vi "art联动采集V4.2.vi"() -> ()   [LabVIEW 2016]
uses:
  <vilib>/Instr/_visa.llb/VISA Configure Serial Port (Instr).vi
  <vilib>/Utility/file.llb/Write Delimited Spreadsheet (DBL).vi
panel:
  in  "定位模式":bool
  in  "X终点":dbl
  in  "Y终点":dbl
  in  "高级设置":bool
  in  "Y轴回零速度":dbl=15000.0
  in  "X轴回零速度":dbl=15000.0
  in  "细分设置":dbl=8.0
  in  "等待时间":u32=40
  in  "文件保存":path=path "C:/Users/H301/Desktop/art采集实验数据" caption="保存路径"
  out "行用时（s）":dbl
  out "time（行）":u32
  out "hDevice out":i32=253955776
  out "error out":errorcluster caption="错误输出"
  in  "退出扫描(Esc)":bool
  out "N_Length":i32=16384
  out "M_Length":i32
  out "hDevice":i32=241832032
  out "pulDDR2Length":u32=256
  out "总用时（s）":dbl
  out "毫秒计时值":u32=3586537
  out "数组":dbl[][](array[numeric])=[[58819.77200735986, 88200.32943600747]]
  out "强度图":dbl[][](graph)=[[58819.77200735986, 88200.32943600747]]
  out "judge":dbl
  out "Xloop":dbl
  out "幅频谱":dbl[](graph)
  out "时域谱":dbl[](graph)
  out "错误输出":errorcluster
  in  "启动":bool
  in  "开始扫描":bool
  in  "X归零":bool
  in  "Y归零":bool
  in  "Y起点":dbl
  in  "Y轴速度":dbl=9000.0
  in  "X轴速度":dbl=9000.0
  out "电机状态":bool
  in  "电机端口":refnum<visa-resource-name>="COM6"
  out "Yloop":dbl=1.0
  out "X扫描范围":dbl=150.0
  out "Y扫描范围":dbl=75.0
  out "Y序":i32
  in  "X起点":dbl
  out "Y(mm)":dbl
  out "x+y 2":dbl=3.0
  in  "Y步进":dbl=1.0
  in  "精度":dbl=0.001
  in  "电机急停":bool
  out "X（mm）":dbl
  out "x+y":dbl=1.0
  in  "X步进":dbl=1.0
  # "实时坐标"
  # "时域谱"
  # "频域谱"
  # "扫描参数"
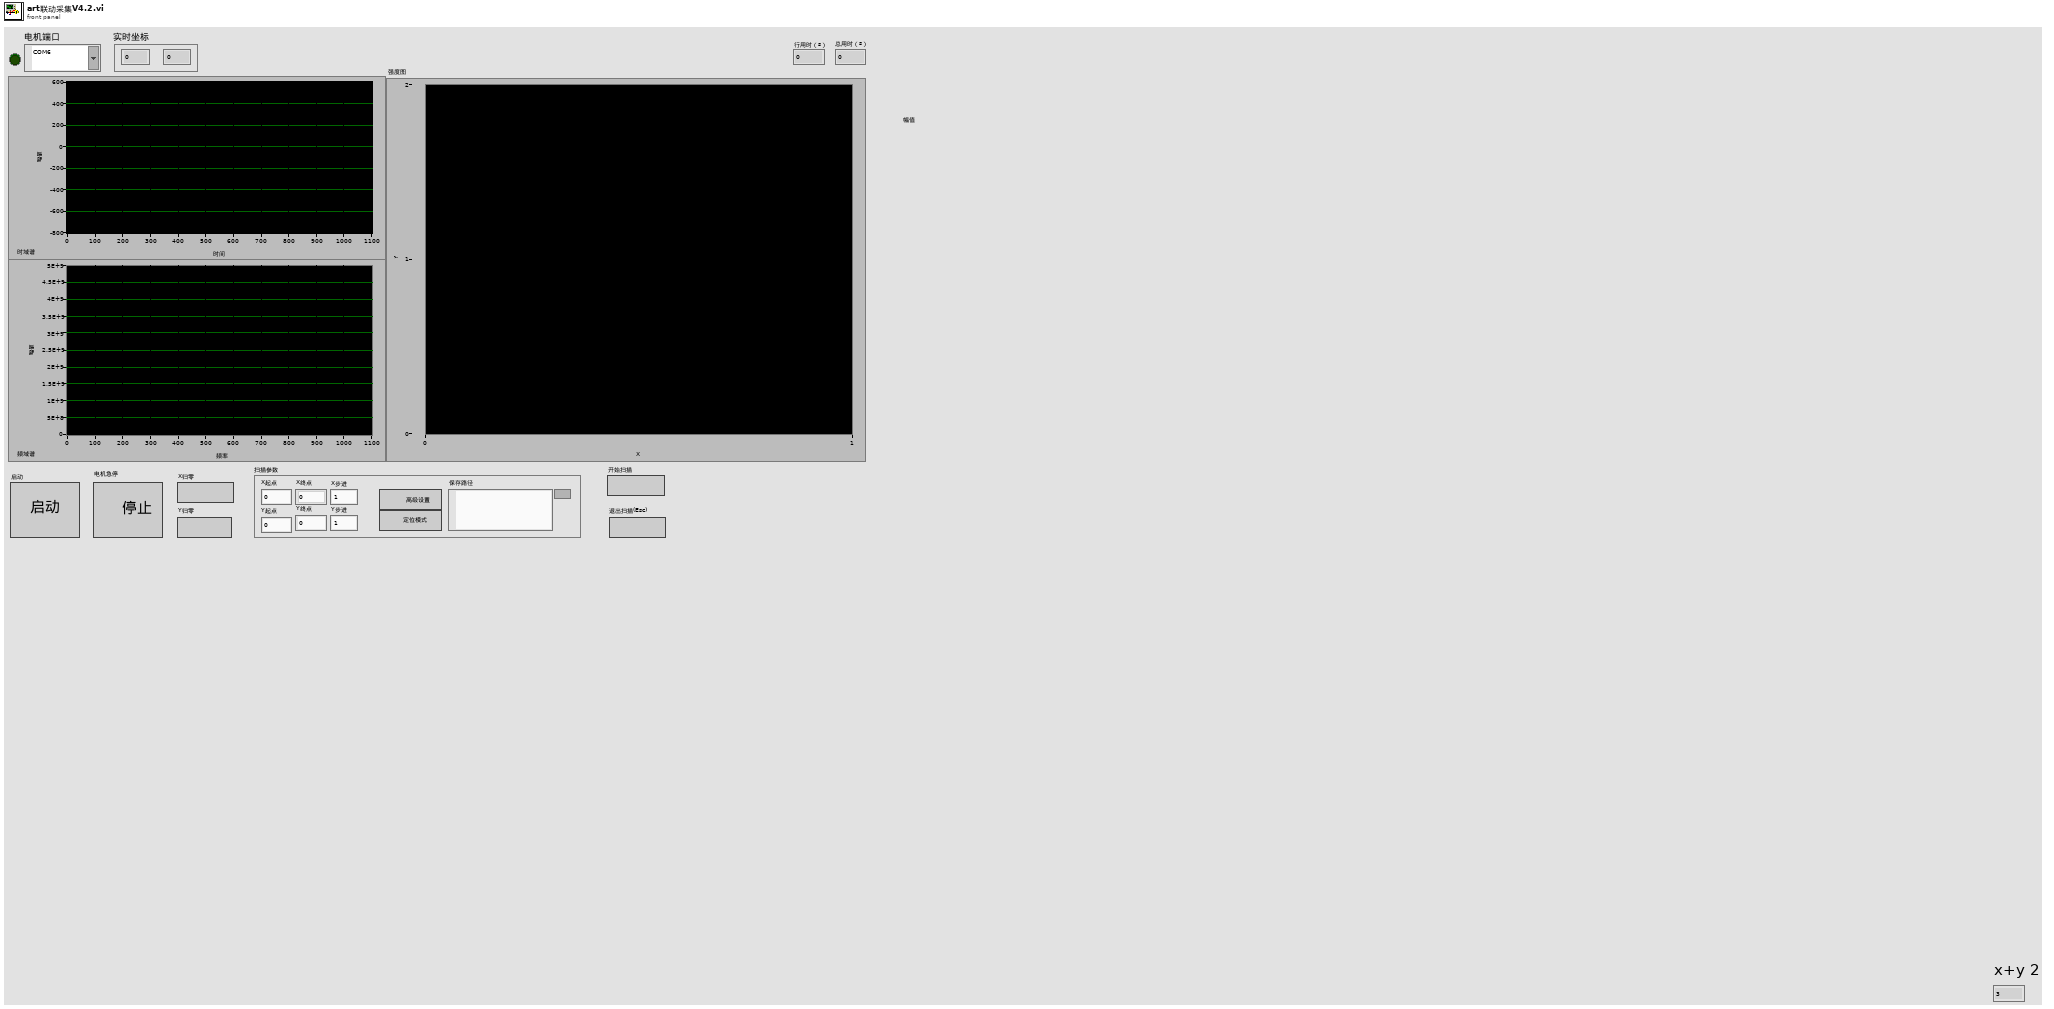
[diagram p1: front panel]
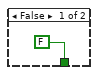
[diagram p2: hidden frame]
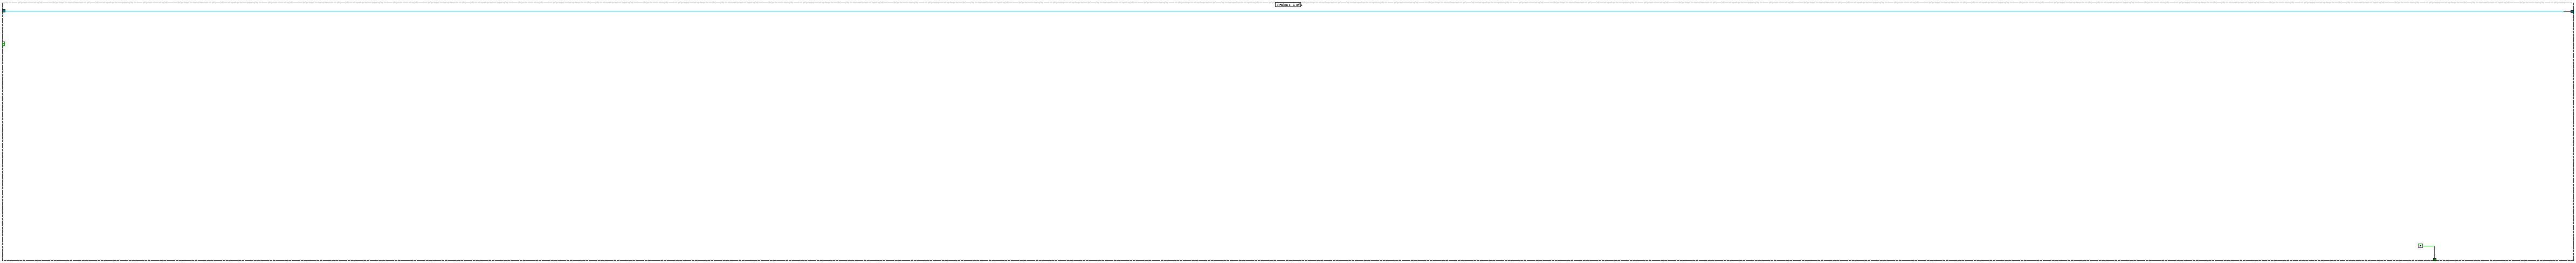
[diagram p3: hidden frame]
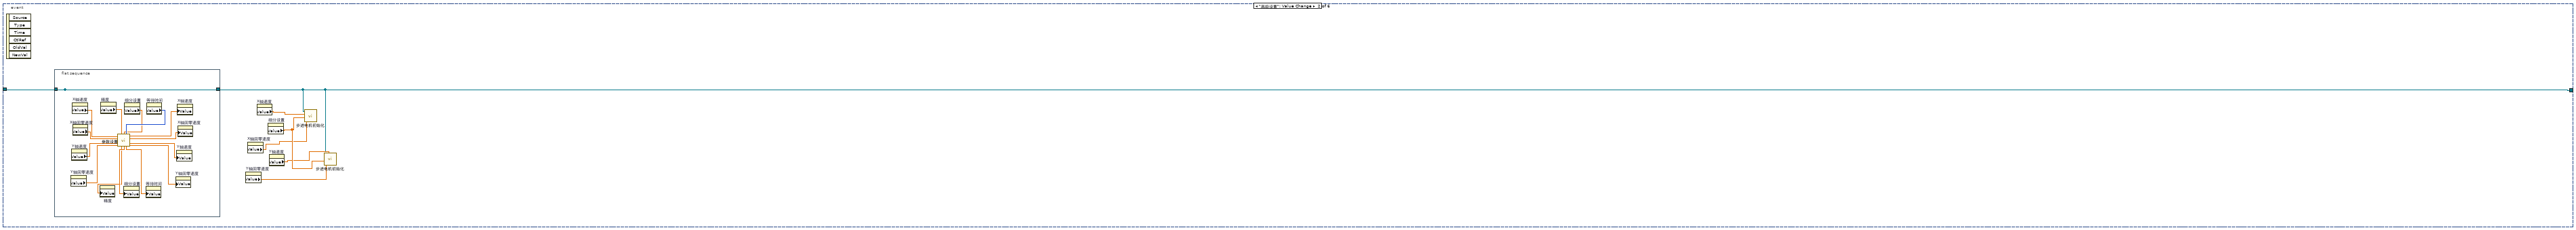
[diagram p4: hidden frame]
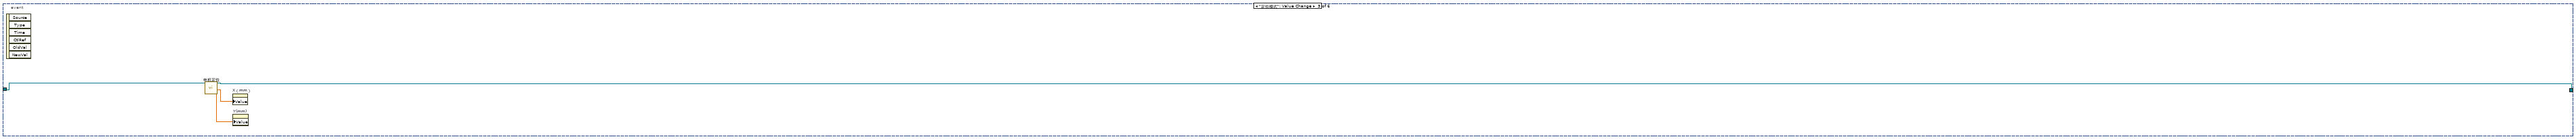
[diagram p5: hidden frame]
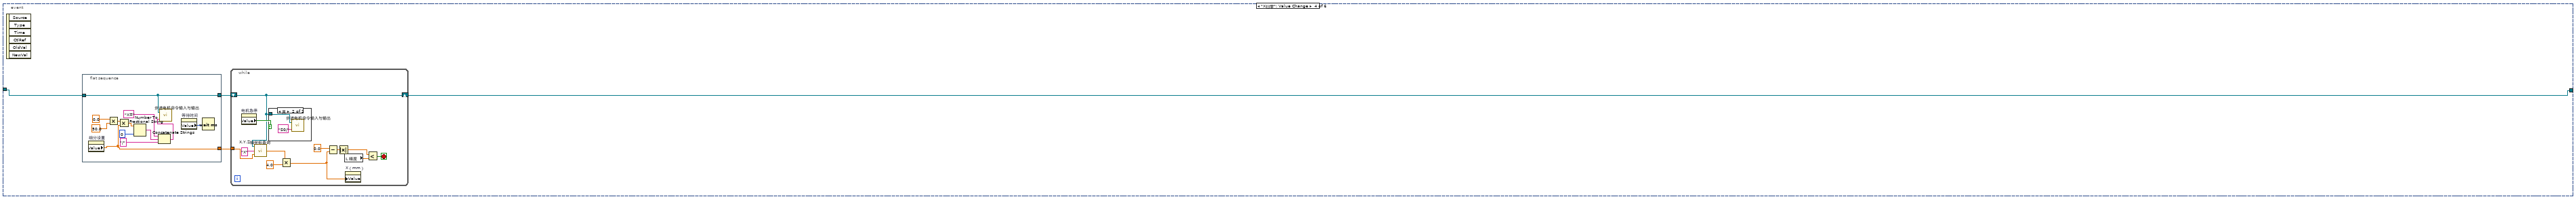
[diagram p6: hidden frame]
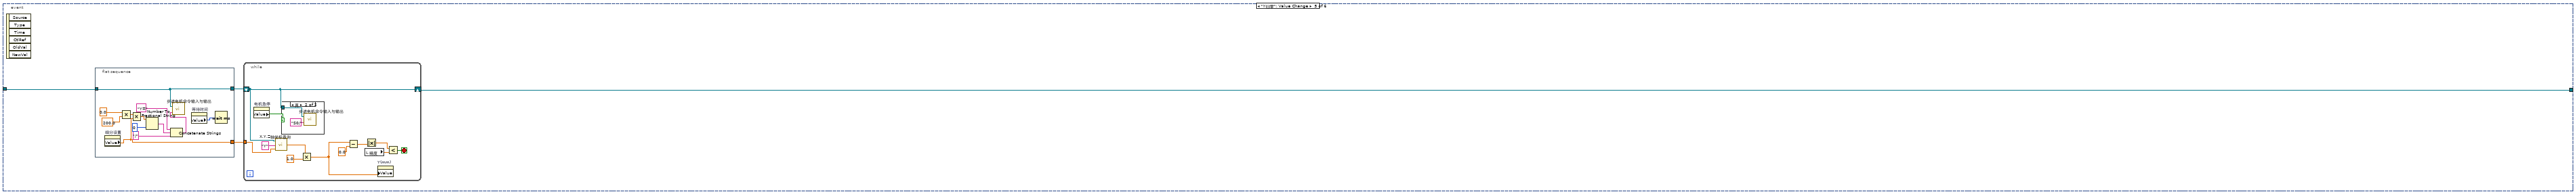
[diagram p8: hidden frame]
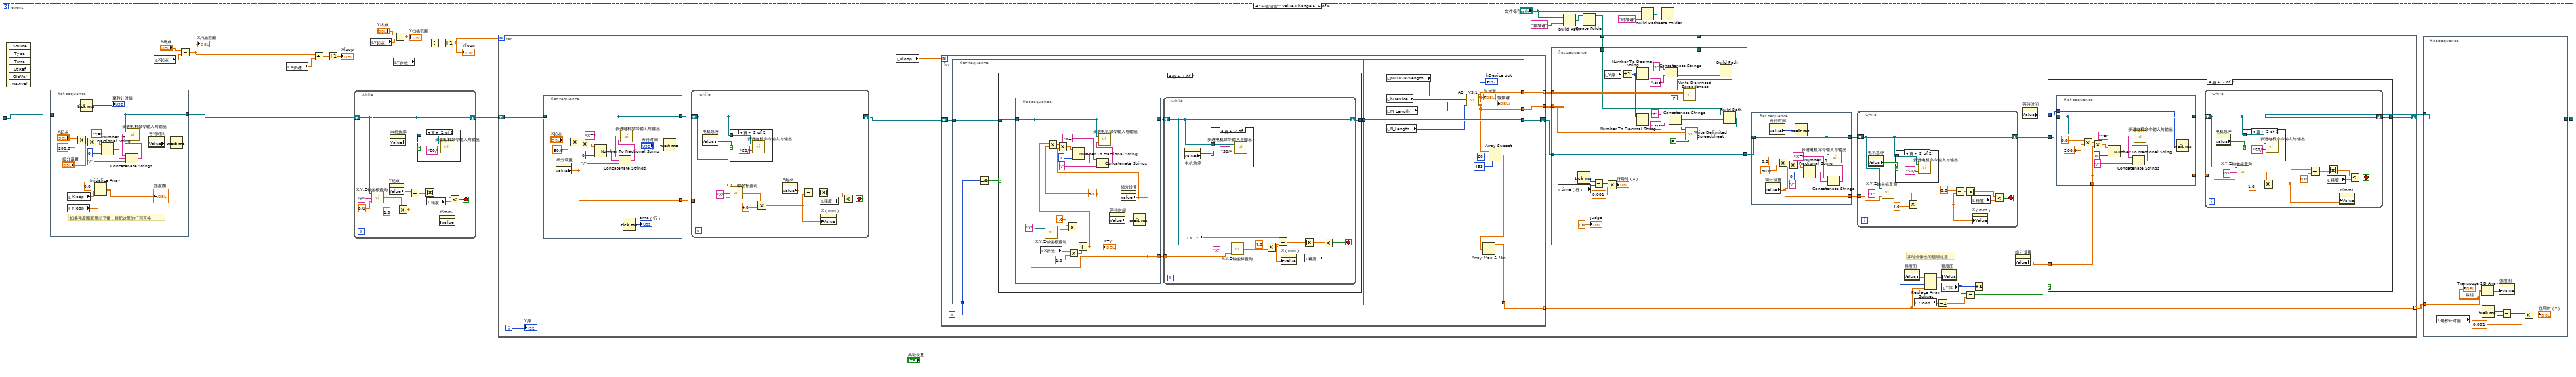
[diagram p10: hidden frame]
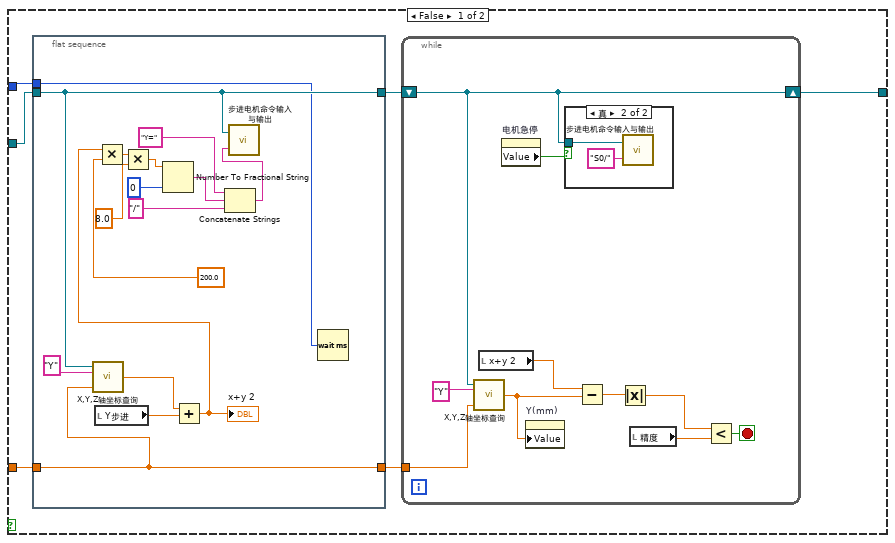
[diagram p14: hidden frame]
diagram:
  n1 = while {
    stop <- w3 stop-if-true
    n2 = case shown="真" "启动" {
      tunnel: [FALSE ("ESC") w10] -> w3
      frame False {
      }
      frame True {
        w25 = 0  # OutClockSource
        w26 = 0  # bClockSourceDir
        w28 = 10000000  # Frequency
        w29 = 0  # ClockSource
        w30 = 0  # TrigLevelVolt
        w17 = 1
        w31 = 0  # TriggerDir
        w32 = 0  # TriggerSource
        w33 = 0  # ATRTriggerChannel
        w34 = 0  # TriggerMode
        w18 = 4096  # N_Length
        w19 = 0  # M_Length
        w35 = 1  # CouplingType
        w36 = 0  # DeviceLgcID
        w46 = u16 0 items=["无", "XON/XOFF", "RTS/CTS", "XON/XOFF & RTS/CTS", "DTR/DSR", "XON/XOFF & DTR/DSR"] ("flow control (0:none)")
        w47 = u16 10 items=["1.0"=10, "1.5"=15, "2.0"=20] ("stop bits (10: 1 bit)")
        # "3"
        # "2"
        # "1"
        n3 = call-poly "VISA Configure Serial Port"("VISA resource name"="电机端口", "baud rate (9600)"=u32 9600, "data bits (8)"=u16 8, "parity (0:none)"=enum16{"None", "Odd", "Even", "Mark", "Space"}."None", "stop bits (10: 1 bit)"=w47, "flow control (0:none)"=w46) -> ("VISA resource name out"=w38:refnum<visa-resource-name>, "error out"=→"error out":errorcluster)  [unwired: 1 in, 7 out]
        n4 = Build Array "InputRange"(w17, w17, w17, w17) -> (w16:i32[])
        n5 = dll-call lib="PTH2aabs CUsersH301Desktopart闭环扫描程序采集卡控制INFamd64PCI8502_32.dll" fn="PCI8502_CreateDevice" label="CreateDevice"("DeviceLgcID"=w36) -> (w23:i32)  [unwired: 4 in, 2 out]
        n6 = property on="细分设置" class="DigNum (严格)"() -> ("Value"=w9:dbl)  [unwired: 2 in, 2 out]
        n7 = Build Array (concatenate) "InitDeviceAD"(w28, w16, w35, w19, w18, w34, w33, w32, w31, w30, w29, w26, w25) -> (w27:i32[])
        n8 = call "步进电机初始化.vi"("回零速度"="X轴回零速度", "细分设置"=w9, "X轴速度"="X轴速度", "串口通信端口"=w38) -> ()  [unwired: 2 in, 1 out]
        n9 = dll-call lib="PTH2aabs CUsersH301Desktopart闭环扫描程序采集卡控制INFamd64PCI8502_32.dll" fn="PCI8502_GetDDR2Length" label="GetDDR2Length"("hDevice"=w23, "pulDDR2Length"=u32 0) -> ("hDevice"=w22:i32, "pulDDR2Length"=→"pulDDR2Length":u32)  [unwired: 4 in, 2 out]
        n10 = call "步进电机初始化.vi"("Y轴速度"="Y轴速度", "回零速度"="Y轴回零速度", "细分设置"=w9, "串口通信端口"=w38) -> ()  [unwired: 2 in, 1 out]
        n11 = call "步进电机命令输入与输出.vi"("输入字符串"="?R/", "串口通信端口"=w38) -> ("返回字符串"=w43:string)
        n12 = dll-call lib="PTH2aabs CUsersH301Desktopart闭环扫描程序采集卡控制INFamd64PCI8502_32.dll" fn="PCI8502_InitDeviceAD" label="InitDeviceAD"("hDevice"=w22, "pADPara"=w27) -> ("hDevice"=→"hDevice":i32)  [unwired: 5 in, 2 out]
        n13 = String Subset(string=w43, offset (0)=0 ("偏移量(0)"), length (rest)=2 ("长度（剩余）")) -> (substring=w40:string)
        n14 = Equal?(x=w40, y="OK") -> (x = y?=w37:bool)
        "电机状态" <- w37
        n15 = case shown="真" w37 {
          tunnel: w38 -> [w53 w56]
          tunnel: [w53 w54] -> w11
          tunnel: [FALSE ("ESC") w55] -> w10
          frame False {
          }
          frame True {
            n16 = while {
              tunnel: ["退出扫描(Esc)"] -> w55
              shift-right: [w57] -> w54
              shift-left: w56 -> [w62]
              stop <- "退出扫描(Esc)" stop-if-true
              n17 = property on="高级设置" class="Bool"("Visible"=TRUE ("可见")) -> ()  [unwired: 2 in, 2 out]
              n18 = property on="定位模式" class="Bool"("Visible"=TRUE ("可见")) -> ()  [unwired: 2 in, 2 out]
              n19 = event shown="[0] 超时" {
                selector: _ -> [_ _ _ _ _ _]
                dyn-events: _ -> [_ _ _ _ _ _]
                timeout: 1 -> [_ _ _ _ _ _]
                tunnel: w62 -> [w63 w70 w89 w93 w123 w174]
                tunnel: [w63 w64 w88 w91 w121 w168] -> w57
                event Timeout {
                  n20 = event-data() -> ()  [unwired: 1 in, 3 out]
                }
                event "高级设置": Value Change {
                  n21 = event-data() -> ()  [unwired: 1 in, 6 out]
                  n22 = flat-sequence {
                    tunnel: w70 -> [w71]
                    tunnel: [w71] -> _
                    tunnel: [w71] -> w64
                    frame #0 {
                      n23 = property on="Y轴回零速度" class="DigNum (严格)"() -> ("Value"=w75:dbl)  [unwired: 2 in, 2 out]
                      n24 = property on="Y轴速度" class="DigNum (严格)"() -> ("Value"=w74:dbl)  [unwired: 2 in, 2 out]
                      n25 = property on="X轴速度" class="DigNum (严格)"() -> ("Value"=w72:dbl)  [unwired: 2 in, 2 out]
                      n26 = property on="X轴回零速度" class="DigNum (严格)"() -> ("Value"=w73:dbl)  [unwired: 2 in, 2 out]
                      n27 = property on="精度" class="DigNum (严格)"() -> ("Value"=w79:dbl)  [unwired: 2 in, 2 out]
                      n28 = property on="细分设置" class="DigNum (严格)"() -> ("Value"=w80:dbl)  [unwired: 2 in, 2 out]
                      n29 = property on="等待时间" class="DigNum (严格)"() -> ("Value"=w81:u32)  [unwired: 2 in, 2 out]
                      n30 = call "参数设置.vi"("X轴速度"=w72, "精度"=w79, "细分设置"=w80, "等待时间"=w81, "X轴回零速度"=w73, "Y轴速度"=w74, "Y轴回零速度"=w75) -> ("X轴速度"=w82:dbl, "X轴回零速度"=w83:dbl, "Y轴速度"=w84:dbl, "精度"=w76:dbl, "细分设置"=w77:dbl, "等待时间"=w78:dbl, "Y轴回零速度"=w85:dbl)  [unwired: 2 in]
                      n31 = property on="精度" class="DigNum (严格)"("Value"=w76) -> ()  [unwired: 2 in, 2 out]
                      n32 = property on="细分设置" class="DigNum (严格)"("Value"=w77) -> ()  [unwired: 2 in, 2 out]
                      n33 = property on="等待时间" class="DigNum (严格)"("Value"=w78) -> ()  [unwired: 2 in, 2 out]
                      n34 = property on="Y轴回零速度" class="DigNum (严格)"("Value"=w85) -> ()  [unwired: 2 in, 2 out]
                      n35 = property on="Y轴速度" class="DigNum (严格)"("Value"=w84) -> ()  [unwired: 2 in, 2 out]
                      n36 = property on="X轴速度" class="DigNum (严格)"("Value"=w82) -> ()  [unwired: 2 in, 2 out]
                      n37 = property on="X轴回零速度" class="DigNum (严格)"("Value"=w83) -> ()  [unwired: 2 in, 2 out]
                    }
                  }
                  n38 = property on="Y轴回零速度" class="DigNum (严格)"() -> ("Value"=w66:dbl)  [unwired: 2 in, 2 out]
                  n39 = property on="X轴回零速度" class="DigNum (严格)"() -> ("Value"=w67:dbl)  [unwired: 2 in, 2 out]
                  n40 = property on="X轴速度" class="DigNum (严格)"() -> ("Value"=w68:dbl)  [unwired: 2 in, 2 out]
                  n41 = property on="细分设置" class="DigNum (严格)"() -> ("Value"=w69:dbl)  [unwired: 2 in, 2 out]
                  n42 = property on="Y轴速度" class="DigNum (严格)"() -> ("Value"=w65:dbl)  [unwired: 2 in, 2 out]
                  n43 = call "步进电机初始化.vi"("回零速度"=w67, "细分设置"=w69, "X轴速度"=w68, "串口通信端口"=w64) -> ()  [unwired: 2 in, 1 out]
                  n44 = call "步进电机初始化.vi"("Y轴速度"=w65, "回零速度"=w66, "细分设置"=w69, "串口通信端口"=w64) -> ()  [unwired: 2 in, 1 out]
                }
                event "定位模式": Value Change {
                  n45 = event-data() -> ()  [unwired: 1 in, 6 out]
                  n46 = call "电机定位.vi"("VISA I"=w89) -> ("Y"=w86:dbl, "X"=w87:dbl, "VISA O"=w88:refnum<visa-resource-name>)  [unwired: 8 in]
                  n47 = property on="X（mm）" class="DigNum (严格)"("Value"=w87) -> ()  [unwired: 2 in, 2 out]
                  n48 = property on="Y(mm)" class="DigNum (严格)"("Value"=w86) -> ()  [unwired: 2 in, 2 out]
                }
                event "X归零": Value Change {
                  n49 = event-data() -> ()  [unwired: 1 in, 6 out]
                  n50 = flat-sequence {
                    tunnel: w93 -> [w97]
                    tunnel: [w97] -> w92
                    tunnel: [w94] -> w90
                    frame #0 {
                      n51 = property on="细分设置" class="DigNum (严格)"() -> ("Value"=w94:dbl)  [unwired: 2 in, 2 out]
                      n52 = Multiply(x=0.0, y=50.0) -> (x*y=w100:dbl)
                      n53 = Multiply(x=w100, y=w94) -> (x*y=w105:dbl)
                      n54 = Number To Fractional String(number=w105, precision (6)=i16 0 ("精度(6)")) -> (F-format string=w103:string)  [unwired: 2 out]
                      n55 = Concatenate Strings("X=" ("字符串"), w103, "/" ("字符串")) -> (w98:string)
                      n56 = call "步进电机命令输入与输出.vi"("输入字符串"=w98, "串口通信端口"=w97) -> ()  [unwired: 1 out]
                      n57 = property on="等待时间" class="DigNum (严格)"() -> ("Value"=w95:u32)  [unwired: 2 in, 2 out]
                      n58 = Wait (ms)(milliseconds to wait=w95) -> ()  [unwired: 1 out]
                    }
                  }
                  n59 = while {
                    tunnel: w90 -> [w106]
                    shift-right: [w107] -> w91
                    shift-left: w92 -> [w107]
                    stop <- w113 stop-if-true
                    n60 = property on="电机急停" class="Bool (严格)"() -> ("Value"=w114:bool)  [unwired: 2 in, 2 out]
                    n61 = call "X,Y,Z轴坐标查询.vi"("细分设置"=w106, "查询坐标轴"="X", "串口通信端口"=w107) -> ("坐标(mm)"=w115:dbl)
                    n62 = case shown="真" w114 {
                      tunnel: w107 -> [_ w118]
                      frame False {
                      }
                      frame True {
                        n63 = call "步进电机命令输入与输出.vi"("输入字符串"="S0/", "串口通信端口"=w118) -> ()  [unwired: 1 out]
                      }
                    }
                    n64 = Multiply(x=w115, y=4.0 ("x")) -> (x*y=w111:dbl)
                    n65 = Subtract(x=0.0, y=w111) -> (x-y=w110:dbl)
                    n66 = Absolute Value(x=w110) -> (abs(x)=w109:dbl)
                    n67 = local read "精度"() -> (w112:dbl)
                    n68 = property on="X（mm）" class="DigNum (严格)"("Value"=w111) -> ()  [unwired: 2 in, 2 out]
                    n69 = Less?(x=w109, y=w112) -> (x < y?=w113:bool)
                  }
                }
                event "Y归零": Value Change {
                  n70 = event-data() -> ()  [unwired: 1 in, 6 out]
                  n71 = flat-sequence {
                    tunnel: w123 -> [w127]
                    tunnel: [w127] -> w122
                    tunnel: [w124] -> w120
                    frame #0 {
                      n72 = property on="细分设置" class="DigNum (严格)"() -> ("Value"=w124:dbl)  [unwired: 2 in, 2 out]
                      n73 = Multiply(x=0.0, y=200.0) -> (x*y=w130:dbl)
                      n74 = Multiply(x=w130, y=w124) -> (x*y=w135:dbl)
                      n75 = Number To Fractional String(number=w135, precision (6)=i16 0 ("精度(6)")) -> (F-format string=w133:string)  [unwired: 2 out]
                      n76 = Concatenate Strings("Y=" ("字符串"), w133, "/" ("字符串")) -> (w128:string)
                      n77 = call "步进电机命令输入与输出.vi"("输入字符串"=w128, "串口通信端口"=w127) -> ()  [unwired: 1 out]
                      n78 = property on="等待时间" class="DigNum (严格)"() -> ("Value"=w125:u32)  [unwired: 2 in, 2 out]
                      n79 = Wait (ms)(milliseconds to wait=w125) -> ()  [unwired: 1 out]
                    }
                  }
                  n80 = while {
                    tunnel: w120 -> [w136]
                    shift-right: [w137] -> w121
                    shift-left: w122 -> [w137]
                    stop <- w143 stop-if-true
                    n81 = property on="电机急停" class="Bool (严格)"() -> ("Value"=w144:bool)  [unwired: 2 in, 2 out]
                    n82 = call "X,Y,Z轴坐标查询.vi"("细分设置"=w136, "查询坐标轴"="Y", "串口通信端口"=w137) -> ("坐标(mm)"=w145:dbl)
                    n83 = case shown="真" w144 {
                      tunnel: w137 -> [_ w148]
                      frame False {
                      }
                      frame True {
                        n84 = call "步进电机命令输入与输出.vi"("输入字符串"="S0/", "串口通信端口"=w148) -> ()  [unwired: 1 out]
                      }
                    }
                    n85 = Multiply(x=w145, y=1.0 ("x")) -> (x*y=w141:dbl)
                    n86 = Subtract(x=w141, y=0.0 ("x")) -> (x-y=w139:dbl)
                    n87 = local read "精度"() -> (w142:dbl)
                    n88 = Absolute Value(x=w139) -> (abs(x)=w138:dbl)
                    n89 = property on="Y(mm)" class="DigNum (严格)"("Value"=w141) -> ()  [unwired: 2 in, 2 out]
                    n90 = Less?(x=w138, y=w142) -> (x < y?=w143:bool)
                  }
                }
                event "开始扫描": Value Change {
                  n91 = event-data() -> ()  [unwired: 1 in, 6 out]
                  n92 = flat-sequence {
                    tunnel: w174 -> [w191]
                    tunnel: [w191] -> w164
                    frame #0 {
                      # "如果强度图那里出了错，就把这里的行列互换"
                      n93 = local read "Xloop"() -> (w186:dbl)
                      n94 = local read "Yloop"() -> (w185:dbl)
                      n95 = Multiply(x="Y起点", y=200.0) -> (x*y=w194:dbl)
                      n96 = Tick Count (ms)() -> (millisecond timer value=→"毫秒计时值":u32)
                      n97 = Multiply(x=w194, y="细分设置") -> (x*y=w199:dbl)
                      n98 = Initialize Array(0.0 ("元素"), w186, w185) -> (→"强度图":dbl[][])
                      n99 = Number To Fractional String(number=w199, precision (6)=i16 0 ("精度(6)")) -> (F-format string=w197:string)  [unwired: 2 out]
                      n100 = Concatenate Strings("Y=" ("字符串"), w197, "/" ("字符串")) -> (w192:string)
                      n101 = call "步进电机命令输入与输出.vi"("输入字符串"=w192, "串口通信端口"=w191) -> ()  [unwired: 1 out]
                      n102 = property on="等待时间" class="DigNum (严格)"() -> ("Value"=w183:u32)  [unwired: 2 in, 2 out]
                      n103 = Wait (ms)(milliseconds to wait=w183) -> ()  [unwired: 1 out]
                    }
                  }
                  n104 = local read "X起点"() -> (w160:dbl)
                  n105 = Subtract(x="X终点", y=w160) -> (x-y=w159:dbl)
                  "X扫描范围" <- w159
                  n106 = local read "X步进"() -> (w167:dbl)
                  n107 = Divide(x=w159, y=w167) -> (x/y=w165:dbl)
                  n108 = Increment(x=w165) -> (x+1=→"Xloop":dbl)
                  n109 = while {
                    shift-right: [w200] -> w150
                    shift-left: w164 -> [w200]
                    stop <- w205 stop-if-true
                    n110 = call "X,Y,Z轴坐标查询.vi"("细分设置"=8.0, "查询坐标轴"="Y", "串口通信端口"=w200) -> ("坐标(mm)"=w207:dbl)
                    n111 = property on="Y起点" class="DigNum (严格)"() -> ("Value"=w209:dbl)  [unwired: 2 in, 2 out]
                    n112 = property on="电机急停" class="Bool (严格)"() -> ("Value"=w206:bool)  [unwired: 2 in, 2 out]
                    n113 = Multiply(x=w207, y=1.0 ("x")) -> (x*y=w203:dbl)
                    n114 = Subtract(x=w209, y=w203) -> (x-y=w202:dbl)
                    n115 = case shown="真" w206 {
                      tunnel: w200 -> [_ w212]
                      frame False {
                      }
                      frame True {
                        n116 = call "步进电机命令输入与输出.vi"("输入字符串"="S0/", "串口通信端口"=w212) -> ()  [unwired: 1 out]
                      }
                    }
                    n117 = Absolute Value(x=w202) -> (abs(x)=w201:dbl)
                    n118 = local read "精度"() -> (w204:dbl)
                    n119 = property on="Y(mm)" class="DigNum (严格)"("Value"=w203) -> ()  [unwired: 2 in, 2 out]
                    n120 = Less?(x=w201, y=w204) -> (x < y?=w205:bool)
                  }
                  n121 = local read "Y起点"() -> (w162:dbl)
                  n122 = local read "Y步进"() -> (w173:dbl)
                  n123 = Subtract(x="Y终点", y=w162) -> (x-y=w158:dbl)
                  "Y扫描范围" <- w158
                  n124 = Divide(x=w158, y=w173) -> (x/y=w172:dbl)
                  n125 = Increment(x=w172) -> (x+1=w171:dbl)
                  "Yloop" <- w171
                  n126 = Build Path(base path="文件保存", name or relative path="频域谱" ("名称或相对路径")) -> (appended path=w155:path)
                  n127 = Create Folder(path (use dialog)=w155) -> (created path=w151:path)  [unwired: 2 in, 2 out]
                  n128 = Build Path(base path="文件保存", name or relative path="时域谱" ("名称或相对路径")) -> (appended path=w157:path)
                  n129 = Create Folder(path (use dialog)=w157) -> (created path=w152:path)  [unwired: 2 in, 2 out]
                  n130 = for {
                    N: w171 -> [_]
                    shift-right: [w236] -> w170
                    shift-left: w150 -> [w216]
                    tunnel: [w218] -> w169 mode=indexing
                    tunnel: w152 -> [w222]
                    tunnel: w151 -> [w221]
                    i -> [w237]
                    # "实时成像出问题调这里"
                    n131 = flat-sequence {
                      tunnel: w216 -> [w294]
                      tunnel: [w294] -> w235
                      tunnel: [w290] -> w226
                      frame #0 {
                        n132 = property on="细分设置" class="DigNum (严格)"() -> ("Value"=w290:dbl)  [unwired: 2 in, 2 out]
                        n133 = Multiply(x="X起点", y=50.0) -> (x*y=w297:dbl)
                        n134 = Multiply(x=w297, y=w290) -> (x*y=w302:dbl)
                        n135 = Number To Fractional String(number=w302, precision (6)=i16 0 ("精度(6)")) -> (F-format string=w300:string)  [unwired: 2 out]
                        n136 = Concatenate Strings("X=" ("字符串"), w300, "/" ("字符串")) -> (w295:string)
                        n137 = call "步进电机命令输入与输出.vi"("输入字符串"=w295, "串口通信端口"=w294) -> ()  [unwired: 1 out]
                        n138 = Tick Count (ms)() -> (millisecond timer value=→"time（行）":u32)
                        n139 = Wait (ms)(milliseconds to wait="等待时间") -> ()  [unwired: 1 out]
                      }
                    }
                    n140 = while {
                      tunnel: w226 -> [w304]
                      shift-right: [w303] -> w214
                      shift-left: w235 -> [w303]
                      stop <- w309 stop-if-true
                      n141 = property on="电机急停" class="Bool (严格)"() -> ("Value"=w310:bool)  [unwired: 2 in, 2 out]
                      n142 = case shown="真" w310 {
                        tunnel: w303 -> [_ w315]
                        frame False {
                        }
                        frame True {
                          n143 = call "步进电机命令输入与输出.vi"("输入字符串"="S0/", "串口通信端口"=w315) -> ()  [unwired: 1 out]
                        }
                      }
                      n144 = call "X,Y,Z轴坐标查询.vi"("细分设置"=w304, "查询坐标轴"="X", "串口通信端口"=w303) -> ("坐标(mm)"=w311:dbl)
                      n145 = Multiply(x=w311, y=4.0 ("x")) -> (x*y=w307:dbl)
                      n146 = property on="X起点" class="DigNum (严格)"() -> ("Value"=w313:dbl)  [unwired: 2 in, 2 out]
                      n147 = Subtract(x=w313, y=w307) -> (x-y=w306:dbl)
                      n148 = Absolute Value(x=w306) -> (abs(x)=w305:dbl)
                      n149 = local read "精度"() -> (w308:dbl)
                      n150 = property on="X（mm）" class="DigNum (严格)"("Value"=w307) -> ()  [unwired: 2 in, 2 out]
                      n151 = Less?(x=w305, y=w308) -> (x < y?=w309:bool)
                    }
                    n152 = local read "Xloop"() -> (w227:dbl)
                    n153 = for {
                      N: w227 -> [_]
                      shift-right: [w388] -> w215
                      shift-left: w214 -> [w383]
                      tunnel: [w387] -> w234 mode=indexing
                      tunnel: [w386] -> w233 mode=indexing
                      tunnel: [w385] -> w218 mode=indexing
                      i -> [w384]
                      n154 = flat-sequence {
                        tunnel: w383 -> [w393]
                        tunnel: [w392] -> w389
                        tunnel: w384 -> [w390]
                        tunnel: [w443] -> w388
                        tunnel: w389 -> [w443]
                        tunnel: [w442] -> w387
                        tunnel: [w441] -> w386
                        tunnel: [w437] -> w385
                        frame #0 {
                          n155 = Equal To 0?(x=w390) -> (x = 0?=w391:bool)
                          n156 = case shown="假" w391 {
                            tunnel: w393 -> [w396 w431]
                            tunnel: [w395 w431] -> w392
                            frame False {
                              n157 = flat-sequence {
                                tunnel: w396 -> [w406]
                                tunnel: [w406] -> w397
                                tunnel: [w398] -> w394
                                frame #0 {
                                n158 = local read "X步进"() -> (w400:dbl)
                                n159 = Multiply(x=w400, y=1.0 ("x")) -> (x*y=w405:dbl)
                                n160 = property on="等待时间" class="DigNum (严格)"() -> ("Value"=w399:u32)  [unwired: 2 in, 2 out]
                                n161 = property on="细分设置" class="DigNum (严格)"() -> ("Value"=w398:dbl)  [unwired: 2 in, 2 out]
                                n162 = call "X,Y,Z轴坐标查询.vi"("细分设置"=w398, "查询坐标轴"="X", "串口通信端口"=w406) -> ("坐标(mm)"=w402:dbl)
                                n163 = Multiply(x=4.0, y=w402) -> (x*y=w401:dbl)
                                n164 = Add(x=w401, y=w405) -> (x+y=w408:dbl)
                                "x+y" <- w408
                                n165 = Multiply(x=w408, y=50.0) -> (x*y=w411:dbl)
                                n166 = Multiply(x=w411, y=w398) -> (x*y=w416:dbl)
                                n167 = Number To Fractional String(number=w416, precision (6)=i16 0 ("精度(6)")) -> (F-format string=w414:string)  [unwired: 2 out]
                                n168 = Concatenate Strings("X=" ("字符串"), w414, "/" ("字符串")) -> (w409:string)
                                n169 = call "步进电机命令输入与输出.vi"("输入字符串"=w409, "串口通信端口"=w406) -> ()  [unwired: 1 out]
                                n170 = Wait (ms)(milliseconds to wait=w399) -> ()  [unwired: 1 out]
                                }
                              }
                              n171 = while {
                                tunnel: w394 -> [w417]
                                shift-right: [w426] -> w395
                                shift-left: w397 -> [w426]
                                stop <- w425 stop-if-true
                                n172 = property on="电机急停" class="Bool (严格)"() -> ("Value"=w423:bool)  [unwired: 2 in, 2 out]
                                n173 = local read "x+y"() -> (w427:dbl)
                                n174 = case shown="真" w423 {
                                tunnel: w426 -> [_ w429]
                                frame False {
                                }
                                frame True {
                                n175 = call "步进电机命令输入与输出.vi"("输入字符串"="S0/", "串口通信端口"=w429) -> ()  [unwired: 1 out]
                                }
                                }
                                n176 = call "X,Y,Z轴坐标查询.vi"("细分设置"=w417, "查询坐标轴"="X", "串口通信端口"=w426) -> ("坐标(mm)"=w421:dbl)
                                n177 = Multiply(x=4.0, y=w421) -> (x*y=w420:dbl)
                                n178 = Subtract(x=w427, y=w420) -> (x-y=w419:dbl)
                                n179 = property on="X（mm）" class="DigNum (严格)"("Value"=w420) -> ()  [unwired: 2 in, 2 out]
                                n180 = Absolute Value(x=w419) -> (abs(x)=w418:dbl)
                                n181 = local read "精度"() -> (w422:dbl)
                                n182 = Less?(x=w418, y=w422) -> (x < y?=w425:bool)
                              }
                            }
                            frame True {
                            }
                          }
                        }
                        frame #1 {
                          n183 = local read "pulDDR2Length"() -> (w436:u32)
                          n184 = local read "hDevice"() -> (w435:i32)
                          n185 = local read "M_Length"() -> (w434:i32)
                          n186 = local read "N_Length"() -> (w433:i32)
                          n187 = call "AD（V3.1）.vi"("N-length"=w433, "M-length"=w434, "hDevice"=w435, "pulDDR2Length"=w436) -> ("幅频谱"=w441:dbl[], "时域谱"=w442:dbl[], "hDevice out"=→"hDevice out":i32)  [unwired: 5 in]
                          "时域谱" <- w442
                          "幅频谱" <- w441
                          n188 = Array Subset(array=w441, index=60 ("索引"), length=453 ("长度")) -> (w438:dbl[])
                          n189 = Array Max & Min(array=w438) -> (max value=w437:dbl)  [unwired: 3 out]
                        }
                      }
                    }
                    n190 = flat-sequence {
                      tunnel: w233 -> [w271]
                      tunnel: w234 -> [w279]
                      tunnel: w215 -> [w288]
                      tunnel: [w288] -> w229
                      tunnel: w222 -> [w266]
                      tunnel: w221 -> [w265]
                      frame #0 {
                        n191 = local read "time（行）"() -> (w287:u32)
                        n192 = Tick Count (ms)() -> (millisecond timer value=w283:u32)
                        n193 = Subtract(x=w283, y=w287) -> (x-y=w286:u32)
                        n194 = local read "Y序"() -> (w267:i32)
                        n195 = Multiply(x=w286, y=0.001) -> (x*y=→"行用时（s）":dbl)
                        n196 = Increment(x=w267) -> (x+1=w268:i32)
                        n197 = Number To Decimal String(number=w268) -> (decimal integer string=w277:string)  [unwired: 1 in]
                        n198 = Number To Decimal String(number=w268) -> (decimal integer string=w276:string)  [unwired: 1 in]
                        n199 = Concatenate Strings("T" ("字符串"), w277, ".txt" ("字符串")) -> (w280:string)
                        n200 = Concatenate Strings("F" ("字符串"), w276, ".txt" ("字符串")) -> (w274:string)
                        n201 = Build Path(base path=w266, name or relative path=w280) -> (appended path=w282:path)
                        n202 = call-poly <vilib>:"Write Delimited Spreadsheet.vi"("file path (dialog if empty)"=w282, "2D data"=w279, "transpose? (no:F)"=FALSE) -> ()  [unwired: 11 in, 2 out]
                        n203 = Build Path(base path=w265, name or relative path=w274) -> (appended path=w272:path)
                        n204 = call-poly <vilib>:"Write Delimited Spreadsheet.vi"("file path (dialog if empty)"=w272, "2D data"=w271, "transpose? (no:F)"=FALSE) -> ()  [unwired: 11 in, 2 out]
                        "judge" <- 1.0
                      }
                    }
                    n205 = flat-sequence {
                      tunnel: w229 -> [w242]
                      tunnel: [w242] -> w230
                      tunnel: [w240] -> w225
                      frame #0 {
                        n206 = property on="细分设置" class="DigNum (严格)"() -> ("Value"=w240:dbl)  [unwired: 2 in, 2 out]
                        n207 = property on="等待时间" class="DigNum (严格)"() -> ("Value"=w239:u32)  [unwired: 2 in, 2 out]
                        n208 = Multiply(x=0.0, y=50.0) -> (x*y=w245:dbl)
                        n209 = Multiply(x=w245, y=w240) -> (x*y=w250:dbl)
                        n210 = Wait (ms)(milliseconds to wait=w239) -> ()  [unwired: 1 out]
                        n211 = Number To Fractional String(number=w250, precision (6)=i16 0 ("精度(6)")) -> (F-format string=w248:string)  [unwired: 2 out]
                        n212 = Concatenate Strings("X=" ("字符串"), w248, "/" ("字符串")) -> (w243:string)
                        n213 = call "步进电机命令输入与输出.vi"("输入字符串"=w243, "串口通信端口"=w242) -> ()  [unwired: 1 out]
                      }
                    }
                    n214 = while {
                      tunnel: w225 -> [w251]
                      shift-right: [w252] -> w228
                      shift-left: w230 -> [w252]
                      stop <- w258 stop-if-true
                      n215 = property on="电机急停" class="Bool (严格)"() -> ("Value"=w259:bool)  [unwired: 2 in, 2 out]
                      n216 = call "X,Y,Z轴坐标查询.vi"("细分设置"=w251, "查询坐标轴"="X", "串口通信端口"=w252) -> ("坐标(mm)"=w260:dbl)
                      n217 = case shown="真" w259 {
                        tunnel: w252 -> [_ w263]
                        frame False {
                        }
                        frame True {
                          n218 = call "步进电机命令输入与输出.vi"("输入字符串"="S0/", "串口通信端口"=w263) -> ()  [unwired: 1 out]
                        }
                      }
                      n219 = Multiply(x=w260, y=4.0 ("x")) -> (x*y=w256:dbl)
                      n220 = Subtract(x=0.0, y=w256) -> (x-y=w255:dbl)
                      n221 = Absolute Value(x=w255) -> (abs(x)=w254:dbl)
                      n222 = local read "精度"() -> (w257:dbl)
                      n223 = property on="X（mm）" class="DigNum (严格)"("Value"=w256) -> ()  [unwired: 2 in, 2 out]
                      n224 = Less?(x=w254, y=w257) -> (x < y?=w258:bool)
                    }
                    n225 = property on="强度图" class="IntGraph (严格)"() -> ("Value"=w219:dbl[][])  [unwired: 2 in, 2 out]
                    n226 = local read "Yloop"() -> (w231:dbl)
                    n227 = Decrement(x=w231) -> (x-1=w232:dbl)
                    n228 = local read "Y序"() -> (w217:i32)
                    n229 = Replace Array Subset(array=w219, new element=w218, index (col)=w217) -> (w220:dbl[][])  [unwired: 1 in]
                    n230 = property on="强度图" class="IntGraph (严格)"("Value"=w220) -> ()  [unwired: 2 in, 2 out]
                    n231 = Equal?(x=w217, y=w232) -> (x = y?=w238:bool)
                    n232 = Increment(x=w217) -> ()  [unwired: 1 out]
                    n233 = property on="细分设置" class="DigNum (严格)"() -> ("Value"=w223:dbl)  [unwired: 2 in, 2 out]
                    n234 = property on="等待时间" class="DigNum (严格)"() -> ("Value"=w224:u32)  [unwired: 2 in, 2 out]
                    n235 = case shown="真" w238 {
                      tunnel: w228 -> [w322 w354]
                      tunnel: [w320 w355] -> w236
                      tunnel: w224 -> [w318 w352]
                      tunnel: w223 -> [w317 w351]
                      frame False {
                        n236 = flat-sequence {
                          tunnel: w322 -> [w325]
                          tunnel: [w325] -> w321
                          tunnel: [w323] -> w319
                          tunnel: w318 -> [w324]
                          tunnel: w317 -> [w323]
                          frame #0 {
                            n237 = call "X,Y,Z轴坐标查询.vi"("细分设置"=w323, "查询坐标轴"="Y", "串口通信端口"=w325) -> ("坐标(mm)"=w327:dbl)
                            n238 = local read "Y步进"() -> (w326:dbl)
                            n239 = Add(x=w327, y=w326) -> (x+y=w329:dbl)
                            "x+y 2" <- w329
                            n240 = Multiply(x=w329, y=200.0) -> (x*y=w333:dbl)
                            n241 = Multiply(x=w333, y=8.0 ("细分设置")) -> (x*y=w338:dbl)
                            n242 = Number To Fractional String(number=w338, precision (6)=i16 0 ("精度(6)")) -> (F-format string=w336:string)  [unwired: 2 out]
                            n243 = Concatenate Strings("Y=" ("字符串"), w336, "/" ("字符串")) -> (w331:string)
                            n244 = call "步进电机命令输入与输出.vi"("输入字符串"=w331, "串口通信端口"=w325) -> ()  [unwired: 1 out]
                            n245 = Wait (ms)(milliseconds to wait=w324) -> ()  [unwired: 1 out]
                          }
                        }
                        n246 = while {
                          tunnel: w319 -> [w339]
                          shift-right: [w340] -> w320
                          shift-left: w321 -> [w340]
                          stop <- w346 stop-if-true
                          n247 = call "X,Y,Z轴坐标查询.vi"("细分设置"=w339, "查询坐标轴"="Y", "串口通信端口"=w340) -> ("坐标(mm)"=w344:dbl)
                          n248 = local read "x+y 2"() -> (w347:dbl)
                          n249 = property on="电机急停" class="Bool (严格)"() -> ("Value"=w343:bool)  [unwired: 2 in, 2 out]
                          n250 = property on="Y(mm)" class="DigNum (严格)"("Value"=w344) -> ()  [unwired: 2 in, 2 out]
                          n251 = case shown="真" w343 {
                            tunnel: w340 -> [_ w349]
                            frame False {
                            }
                            frame True {
                              n252 = call "步进电机命令输入与输出.vi"("输入字符串"="S0/", "串口通信端口"=w349) -> ()  [unwired: 1 out]
                            }
                          }
                          n253 = Subtract(x=w347, y=w344) -> (x-y=w342:dbl)
                          n254 = Absolute Value(x=w342) -> (abs(x)=w341:dbl)
                          n255 = local read "精度"() -> (w345:dbl)
                          n256 = Less?(x=w341, y=w345) -> (x < y?=w346:bool)
                        }
                      }
                      frame True {
                        n257 = flat-sequence {
                          tunnel: [w359] -> _
                          tunnel: [w359] -> w356
                          tunnel: w354 -> [w359]
                          tunnel: [w357] -> w353
                          tunnel: w352 -> [w358]
                          tunnel: w351 -> [w357]
                          frame #0 {
                            n258 = Multiply(x=0.0, y=200.0) -> (x*y=w363:dbl)
                            n259 = Multiply(x=w363, y=w357) -> (x*y=w368:dbl)
                            n260 = Number To Fractional String(number=w368, precision (6)=i16 0 ("精度(6)")) -> (F-format string=w366:string)  [unwired: 2 out]
                            n261 = Concatenate Strings("Y=" ("字符串"), w366, "/" ("字符串")) -> (w361:string)
                            n262 = call "步进电机命令输入与输出.vi"("输入字符串"=w361, "串口通信端口"=w359) -> ()  [unwired: 1 out]
                            n263 = Wait (ms)(milliseconds to wait=w358) -> ()  [unwired: 1 out]
                          }
                        }
                        n264 = while {
                          tunnel: w353 -> [w369]
                          shift-right: [w370] -> w355
                          shift-left: w356 -> [w370]
                          stop <- w376 stop-if-true
                          n265 = property on="电机急停" class="Bool (严格)"() -> ("Value"=w377:bool)  [unwired: 2 in, 2 out]
                          n266 = call "X,Y,Z轴坐标查询.vi"("细分设置"=w369, "查询坐标轴"="Y", "串口通信端口"=w370) -> ("坐标(mm)"=w378:dbl)
                          n267 = case shown="真" w377 {
                            tunnel: w370 -> [_ w381]
                            frame False {
                            }
                            frame True {
                              n268 = call "步进电机命令输入与输出.vi"("输入字符串"="S0/", "串口通信端口"=w381) -> ()  [unwired: 1 out]
                            }
                          }
                          n269 = Multiply(x=w378, y=1.0 ("x")) -> (x*y=w374:dbl)
                          n270 = Subtract(x=w374, y=0.0 ("x")) -> (x-y=w372:dbl)
                          n271 = local read "精度"() -> (w375:dbl)
                          n272 = Absolute Value(x=w372) -> (abs(x)=w371:dbl)
                          n273 = property on="Y(mm)" class="DigNum (严格)"("Value"=w374) -> ()  [unwired: 2 in, 2 out]
                          n274 = Less?(x=w371, y=w375) -> (x < y?=w376:bool)
                        }
                      }
                    }
                    "Y序" <- w237
                  }
                  n275 = flat-sequence {
                    tunnel: w170 -> [w177]
                    tunnel: w169 -> [w176]
                    tunnel: [w177] -> w168
                    frame #0 {
                      n276 = local read "毫秒计时值"() -> (w181:u32)
                      n277 = Transpose 2D Array(2D array=w176) -> (transposed array=w175:dbl[][])
                      n278 = Tick Count (ms)() -> (millisecond timer value=w182:u32)
                      n279 = property on="强度图" class="IntGraph (严格)"("Value"=w175) -> ()  [unwired: 2 in, 2 out]
                      n280 = Subtract(x=w182, y=w181) -> (x-y=w178:u32)
                      n281 = Multiply(x=w178, y=0.001) -> (x*y=→"总用时（s）":dbl)
                      "数组" <- w176
                    }
                  }
                }
              }
            }
          }
        }
        n282 = local read "hDevice out"() -> (w14:i32)
        n283 = dll-call lib="PTH2]abs CUsersH301Desktopart闭环扫描程序采集卡控制INFamd64\nPCI8502_32" fn="PCI8502_ReleaseDeviceAD" label="ReleaseDeviceAD"("hDevice"=w14) -> ("hDevice"=w13:i32)  [unwired: 4 in, 2 out]
        n284 = VISA Close(VISA resource name=w11) -> (error out=→"错误输出":errorcluster)  [unwired: 1 in]
        n285 = dll-call lib="PTH2]abs CUsersH301Desktopart闭环扫描程序采集卡控制INFamd64\nPCI8502_32" fn="PCI8502_ReleaseDevice" label="ReleaseDevice"("hDevice"=w13) -> ()  [unwired: 5 in, 2 out]
        "M_Length" <- w19
        "N_Length" <- w18
      }
    }
  }
  n286 = property on="高级设置" class="Bool"("Visible"=FALSE ("可见")) -> ()  [unwired: 2 in, 2 out]
  n287 = property on="定位模式" class="Bool"("Visible"=FALSE ("可见")) -> ()  [unwired: 2 in, 2 out]
